vi "Write Difftrack.lvclass.vi"(8 "error in (no error)":errorcluster, 10 "Difftrack.lvclass":refnum<class "Difftrack.lvclass">, 11 "TargetDef.lvclass in":refnum<class "TargetDef.lvclass">) -> (0 "error out":errorcluster, 3 "TargetDef.lvclass out":refnum<class "TargetDef.lvclass">)   [LabVIEW 2009]
uses:
  TargetDef/TargetDef.lvclass
  Difftrack.lvclass
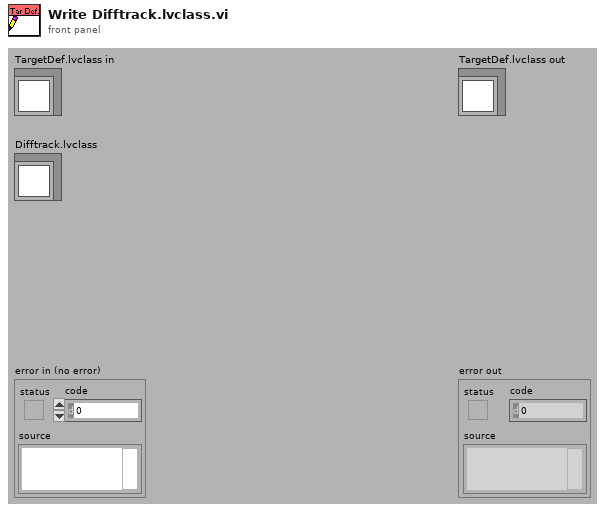
[diagram p1: front panel]
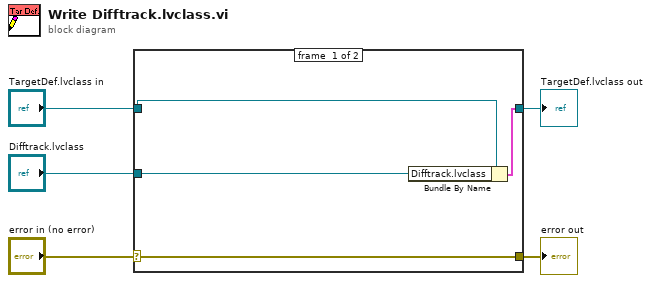
[diagram p0: block diagram]
diagram:
  n1 = case shown="No Error" "error in (no error)" {
    selector: "error in (no error)" -> [w9 w10]
    tunnel: [w9 w10] -> w4
    tunnel: [w7 w11] -> w2
    tunnel: "TargetDef.lvclass in" -> [w8 w11]
    tunnel: "Difftrack.lvclass" -> [w6 _]
    frame #0 {
      n2 = Bundle By Name(cluster=w8, "Difftrack.lvclass"=w6) -> (w7:cluster{})
    }
    frame #1 {
    }
  }
  "error out" <- w4
  "TargetDef.lvclass out" <- w2
